vi "Queue Comms FGV.vi"(8 "error in (no error)":errorcluster, 10 "Action (Get)":T1, 11 "Queue in":refnum<queue>) -> (0 "error out":errorcluster, 3 "Queue out":refnum<queue>)   [LabVIEW 2018, in "Testing UI 2.lvlib"]
doc: "This FGV gets, sets, and releases the communications queue. This communication protocol can easily be switched out for a different communication method.\n\nDefault action is \"Get\" which outputs the queue reference."
uses:
  Testing UI 2.lvlib
  Private Controls/Module Data.ctl
  Private Controls/Module Action.ctl
  Private Controls/Queue Comms FGV Action.ctl
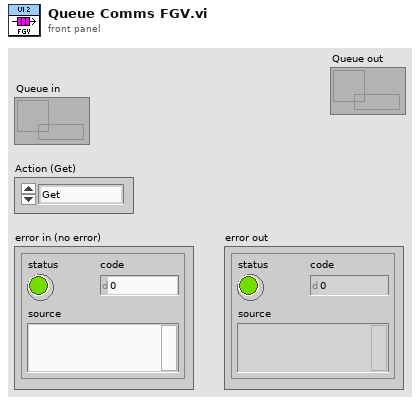
[diagram p1: front panel]
types:
  T1 = typedef "Testing UI 2.lvlib/Queue Comms FGV Action.ctl" = enum16{"Get", "Set", "Release"}
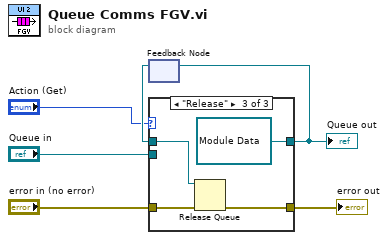
[diagram p0: block diagram]
diagram:
  n1 = feedback #1() -> (w5:refnum<queue>)  [unwired: 1 in]
  n2 = case shown="\"Release\"" "Action (Get)" {
    tunnel: "Queue in" -> [_ w10 _]
    tunnel: "error in (no error)" -> [w7 w9 w13]
    tunnel: w5 -> [w8 _ w14]
    tunnel: [w8 w10 refnum<queue> refnum ("queue out")] -> w4
    tunnel: [w7 w9 w12] -> w6
    frame "Get", Default {
    }
    frame "Set" {
    }
    frame "Release" {
      n3 = Release Queue(queue=w14, error in (no error)=w13) -> (error out=w12:errorcluster)  [unwired: 1 in, 2 out]
    }
  }
  "error out" <- w6
  "Queue out" <- w4
  n4 = feedback-in #1(w4) -> ()
